vi "New Timing Error.vi"(7 "error source vi name":string, 11 "error":T1) -> (1 "new offset":i32, 3 "error out":errorcluster)   [LabVIEW 2017, in "DSF Core.lvlib" / "Timing.lvclass"]
uses:
  Timing.lvclass
  Errors.ctl
  VIs/Constants/Engine Library Name.vi
  LabVIEW-Memory/Source/VIs/New Error Cluster (512B).vi
  LabVIEW-Memory/Source/Static Error Handling.lvlib
  DSF Core.lvlib
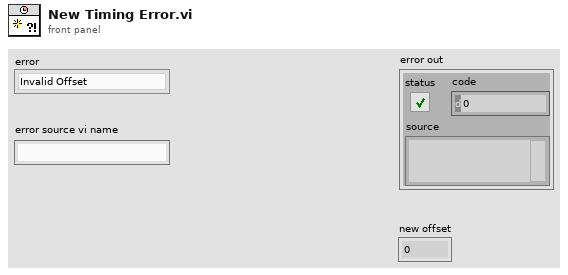
[diagram p1: front panel]
types:
  T1 = typedef "DSF Core.lvlib/Timing.lvclass/Errors.ctl" = enum16{"Invalid Offset", "Invalid Priority"}
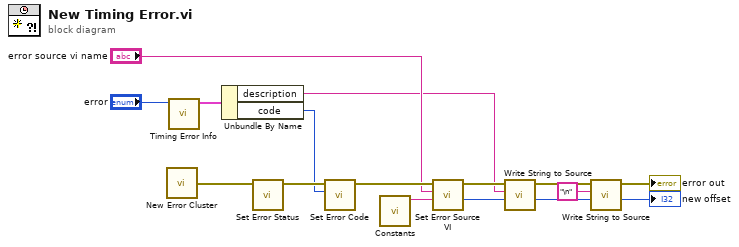
[diagram p0: block diagram]
diagram:
  n1 = call-poly "New Error Cluster.vi"() -> ("error out"=w15:errorcluster)  [unwired: 1 in]
  n2 = call "Timing Error Info.vi"("error"="error") -> ("error info"=w13:cluster{"code":i32, "description":string})  [unwired: 10 in]
  n3 = Unbundle By Name(w13) -> ("description"=w6:string, "code"=w12:i32)
  n4 = call "Set Error Status.vi"("error in"=w15) -> ("error out"=w14:errorcluster)  [unwired: 10 in]
  n5 = call "Set Error Code.vi"("code"=w12, "error in"=w14) -> ("error out"=w11:errorcluster)  [unwired: 9 in]
  n6 = call-poly "Constants.vi"() -> ("Engine Library Name"=w9:string)  [unwired: 11 in]
  n7 = call "Set Error Source VI.vi"("library name (\"\")"=w9, "vi name"="error source vi name", "error in"=w11) -> ("new offset"=w7:i32, "error out"=w8:errorcluster)  [unwired: 7 in]
  n8 = call "Write String to Source.vi"("offset"=w7, "string"=w6, "error in"=w8) -> ("new offset"=w3:i32, "error out"=w5:errorcluster)  [unwired: 7 in]
  n9 = call "Write String to Source.vi"("offset"=w3, "string"="\n", "error in"=w5) -> ("new offset"=→"new offset":i32, "error out"=→"error out":errorcluster)  [unwired: 7 in]
